vi "飽和水蒸気圧.vi"(1 "温度":dbl) -> (0 "飽和水蒸気圧(Pa)":dbl)   [LabVIEW 2014]
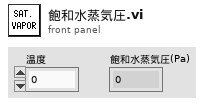
[diagram p1: front panel]
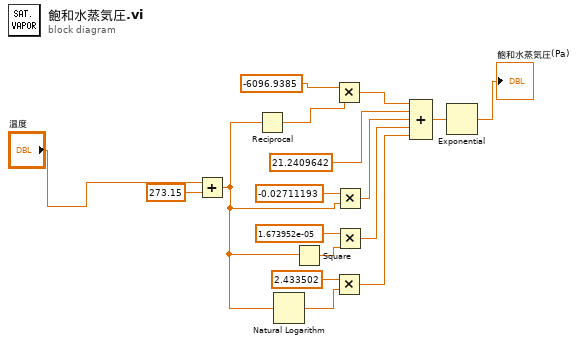
[diagram p0: block diagram]
diagram:
  n1 = Add(x="温度", y=273.15) -> (x+y=w16:dbl)
  n2 = Reciprocal(x=w16) -> (1/x=w7:dbl)
  n3 = Natural Logarithm(1:w16) -> (0:w9:dbl)
  n4 = Square(x=w16) -> (x^2=w6:dbl)
  n5 = Multiply(x=-6096.9385, y=w7) -> (x*y=w10:dbl)
  n6 = Multiply(x=2.433502, y=w9) -> (x*y=w14:dbl)
  n7 = Multiply(x=-0.02711193, y=w16) -> (x*y=w12:dbl)
  n8 = Multiply(x=1.673952e-05, y=w6) -> (x*y=w13:dbl)
  n9 = Compound Arithmetic op=ADD(w10, 21.2409642 ("x"), w12, w13, w14) -> (w15:dbl)
  n10 = Exponential(1:w15) -> (0:→"飽和水蒸気圧(Pa)":dbl)
